vi "PSD_.vi"(10 "Datos":dbl[](array[numeric]), 11 "Frecuencia":dbl) -> (3 "PSD":cluster{"Frecuencia":dbl[], "Amplitud":dbl[]})   [LabVIEW 2012]
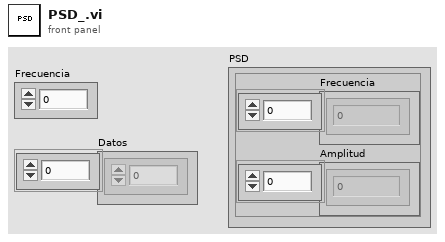
[diagram p1: front panel]
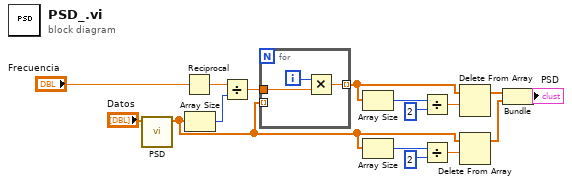
[diagram p0: block diagram]
diagram:
  n1 = call "PSD.vi"("Array in"="Datos") -> ("Array out"=w15:dbl[])  [unwired: 10 in]
  n2 = Reciprocal(x="Frecuencia") -> (1/x=w5:dbl)
  n3 = Array Size(array=w15) -> (size(s)=w1:i32)
  n4 = Divide(x=w5, y=w1) -> (x/y=w2:dbl)
  n5 = for {
    tunnel: w15 -> [_] mode=indexing
    tunnel: w2 -> [w18]
    tunnel: [w17] -> w7 mode=indexing
    i -> [w19]
    n6 = Multiply(x=w19, y=w18) -> (x*y=w17:dbl)
  }
  n7 = Array Size(array=w7) -> (size(s)=w8:i32)
  n8 = Array Size(array=w15) -> (size(s)=w14:i32)
  n9 = Divide(x=w8, y=2) -> (x/y=w10:dbl)
  n10 = Divide(x=w14, y=2) -> (x/y=w12:dbl)
  n11 = Delete From Array(array=w7, length=w10) -> (array with subset deleted=w11:dbl[])  [unwired: 1 in, 1 out]
  n12 = Delete From Array(array=w15, length=w12) -> (array with subset deleted=w16:dbl[])  [unwired: 1 in, 1 out]
  n13 = Bundle(w11, "Array out"=w16) -> (→"PSD":cluster{dbl[], "Array out":dbl[]})  [unwired: 1 in]
